vi "Ramp.vi"(4 "Reinit":bool, 6 "dT (s)":dbl, 10 "Seconds to 1 Unit":dbl, 11 "Input":dbl) -> (3 "Output":dbl)   [LabVIEW 2020]
panel:
  # "Make sure we don't accelerate too fast"
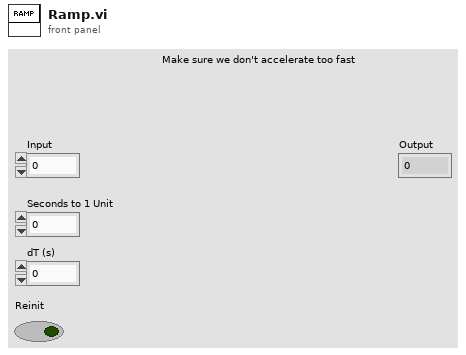
[diagram p1: front panel]
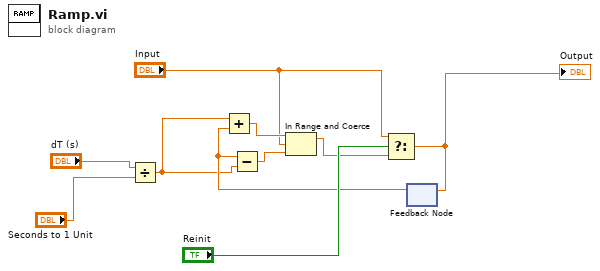
[diagram p0: block diagram]
diagram:
  n1 = Divide(x="dT (s)", y="Seconds to 1 Unit") -> (x/y=w6:dbl)
  n2 = feedback #1() -> (w7:dbl)  [unwired: 1 in]
  n3 = Add(x=w6, y=w7) -> (x+y=w8:dbl)
  n4 = Subtract(x=w7, y=w6) -> (x-y=w5:dbl)
  n5 = In Range and Coerce(upper limit=w8, x="Input", lower limit=w5) -> (coerced(x)=w3:dbl)  [unwired: 1 out]
  n6 = Select(t="Input", s="Reinit", f=w3) -> (s? t:f=w9:dbl)
  "Output" <- w9
  n7 = feedback-in #1(w9) -> ()
